vi "data_load_display_trend_fft_mea_coll_pred_v6.vi"() -> ()   [LabVIEW 2020]
uses:
  <vilib>/Utility/file.llb/Read Delimited Spreadsheet (DBL).vi
panel:
  out "truth vs prediction vs error":dbl[][](graph)
  out "Input vs prediction":dbl[][](graph)
  out "Time vs Acceleration ( Input learning length)":cluster{dbl[], dbl[]}[](graph)
  out "truth vs prediction":dbl[][](graph)
  out "Spectrum plot 2":cluster{i32, dbl, "spectrum out":dbl[]}(graph)
  out "Frequency Interval: delta(f) 2":dbl
  out "xf (frequency) 2":dbl[](array[numeric])
  out "size(s) 2":i32
  out "df (Hz) 2":dbl
  out "ploted signal from each selected frequency 2":dbl[][](graph)
  out "phase 3":dbl[](array[numeric])
  out "magnitude 3":dbl[](array[numeric])
  out "Time vs Acceleration graph(whole data)":cluster{"all rows":dbl[], "all rows":dbl[]}(graph)
  out "Acceleration 2":dbl[](array[numeric])
  out "time 2":dbl[](array[numeric])
  out "array w/ subset deleted 2":dbl[][](array[numeric])
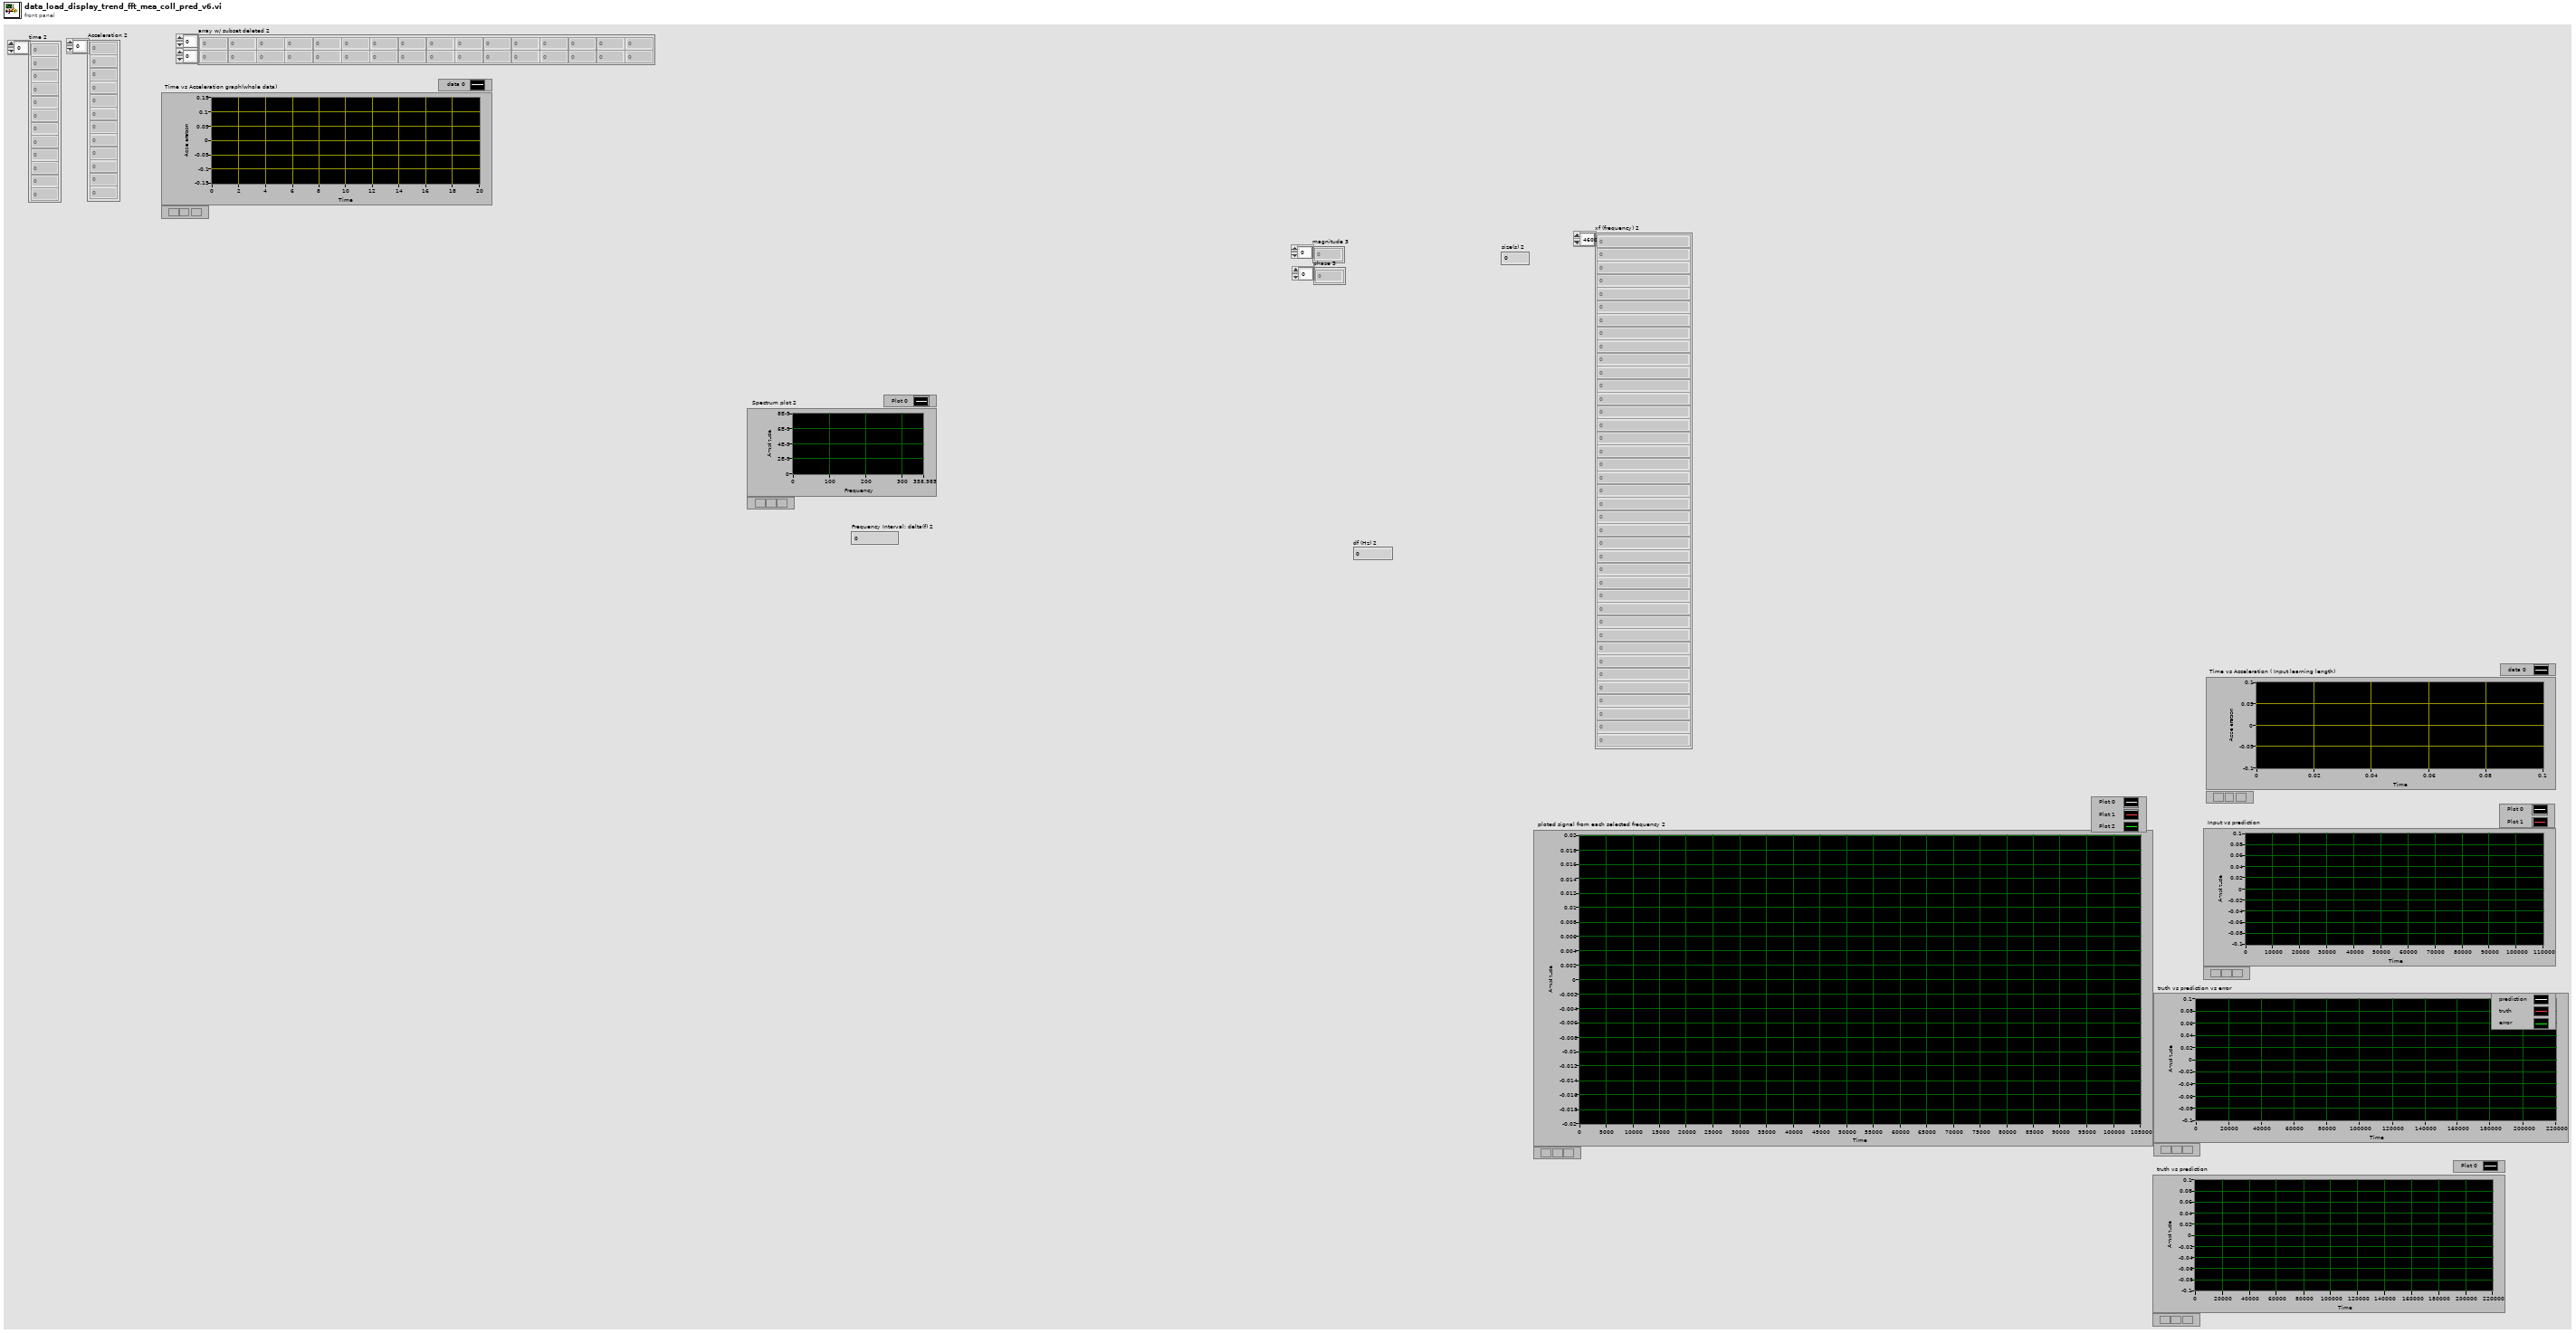
[diagram p1: front panel]
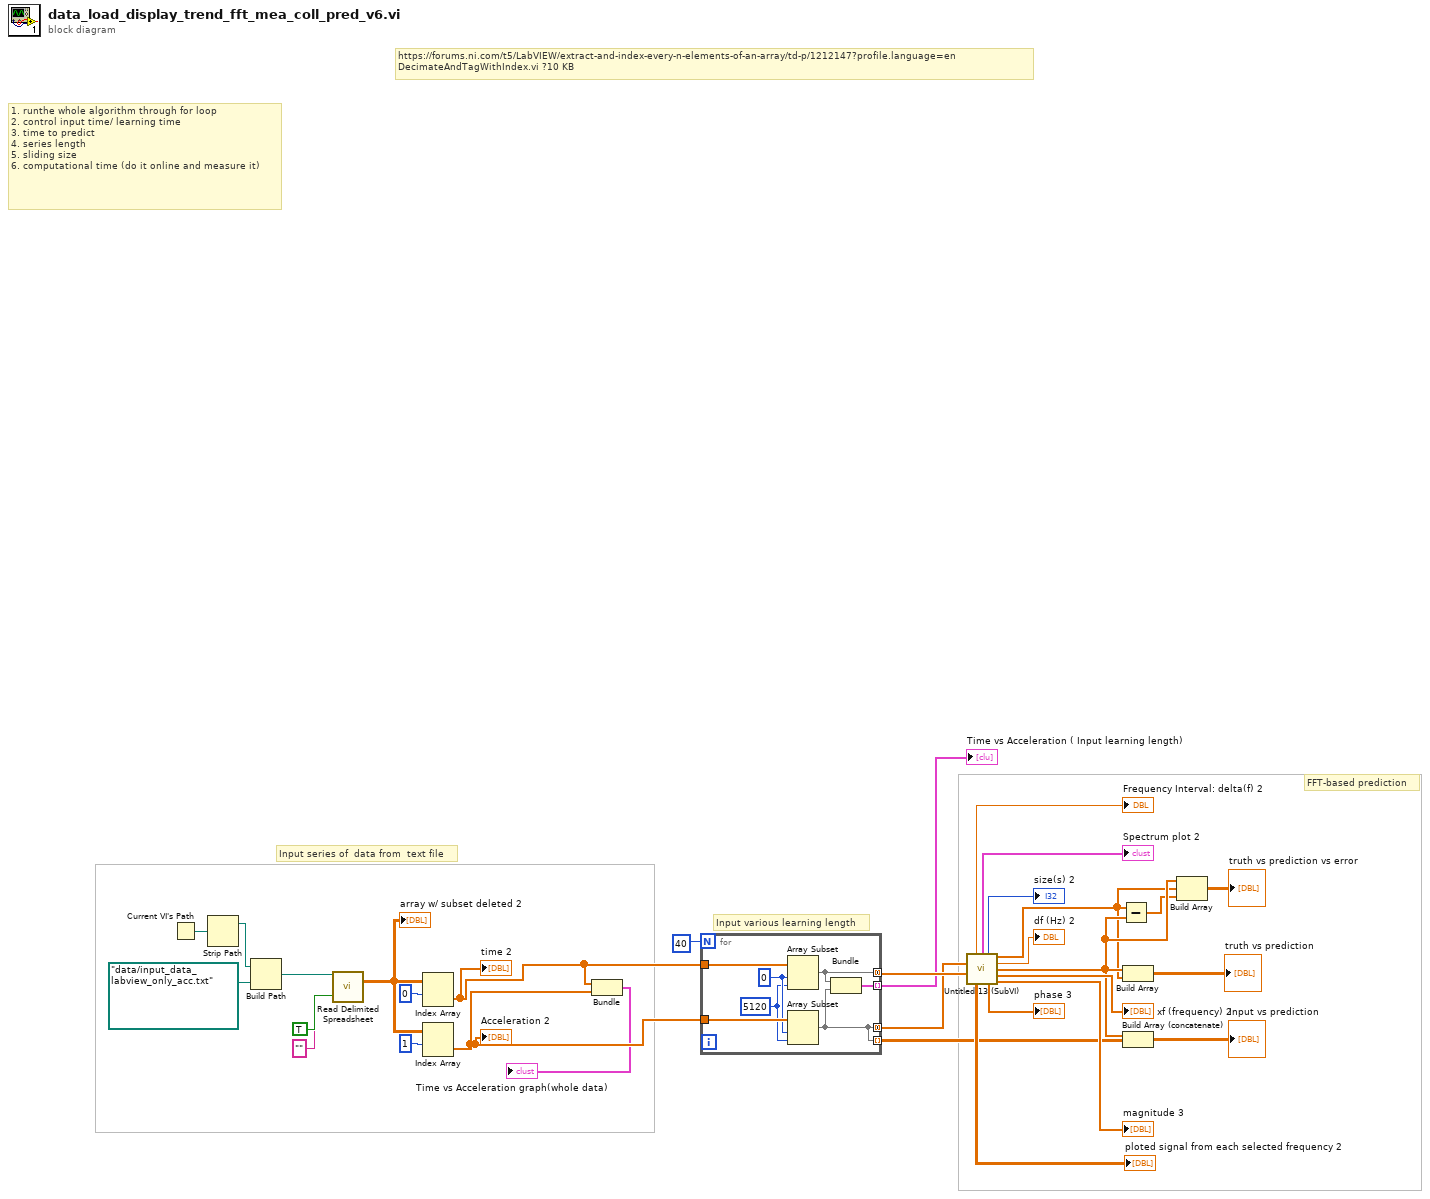
[diagram p0: block diagram]
diagram:
  # "Input series of  data from  text file"
  # "Input various learning length"
  # "FFT-based prediction"
  # "1. runthe whole algorithm through for loop \n2. control input time/ learning time\n3. time to predict\n4. series length\n5. sliding size\n6. computational time (do it online and measure it)"
  # "https://forums.ni.com/t5/LabVIEW/extract-and-index-every-n-elements-of-an-array/td-p/1212147?profile.language=en\nDecimateAndTagWithIndex.vi ?10 KB"
  n1 = Current VI's Path() -> (path=w29:path)
  n2 = Strip Path(path=w29) -> (stripped path=w30:path)  [unwired: 1 out]
  n3 = Build Path(base path=w30, name or relative path=path "data/input_data_labview_only_acc.txt") -> (appended path=w31:path)
  n4 = call-poly <vilib>:"Read Delimited Spreadsheet.vi"("file path (dialog if empty)"=w31, "transpose? (F)"=TRUE, "delimiter (\\t)"="" ("delimiter (\\t)")) -> ("all rows"=w28:dbl[][])  [unwired: 7 in, 5 out]
  "array w/ subset deleted 2" <- w28
  n5 = Index Array(array=w28, index (row)=0) -> (element=w13:dbl[])  [unwired: 1 in]
  "time 2" <- w13
  n6 = Index Array(array=w28, index (row)=1) -> (element=w11:dbl[])  [unwired: 1 in]
  "Acceleration 2" <- w11
  n7 = Bundle("all rows"=w13, "all rows"=w11) -> (→"Time vs Acceleration graph(whole data)":cluster{"all rows":dbl[], "all rows":dbl[]})  [unwired: 1 in]
  n8 = for {
    N: 40 -> [_]
    tunnel: w13 -> [w38]
    tunnel: [w35] -> w10 mode=concatenating
    tunnel: w11 -> [w37]
    tunnel: [w33] -> w9 mode=concatenating
    tunnel: [w34] -> w8 mode=indexing
    tunnel: [w33] -> w7 mode=indexing
    w36 = 0
    w32 = 5120 ("length")
    n9 = Array Subset(array=w38, index=w36, length=w32) -> (w35:dbl[])
    n10 = Array Subset(array=w37, index=w36, length=w32) -> (w33:dbl[])
    n11 = Bundle(w35, w33) -> (w34:cluster{dbl[], dbl[]})  [unwired: 1 in]
  }
  "Time vs Acceleration ( Input learning length)" <- w8
  n12 = call "Untitled 13 (SubVI).vi"("time"=w10, "acceleration"=w9) -> ("Frequency Interval: delta(f)"=→"Frequency Interval: delta(f) 2":dbl, "Spectrum plot"=→"Spectrum plot 2":cluster{i32, dbl, "spectrum out":dbl[]}, "size(s)"=→"size(s) 2":i32, "all rows"=w4:dbl[], "df (Hz)"=→"df (Hz) 2":dbl, "Array"=w5:dbl[], "xf (frequency)"=→"xf (frequency) 2":dbl[], "ploted signal from each selected frequency"=→"ploted signal from each selected frequency 2":dbl[][], "phase 2"=→"phase 3":dbl[], "magnitude 2"=→"magnitude 3":dbl[])  [unwired: 4 in]
  n13 = Subtract(x=w4, y=w5) -> (x-y=w3:dbl[])
  n14 = Build Array(w5, w4) -> (→"truth vs prediction":dbl[][])
  n15 = Build Array (concatenate)(w5, w7) -> (→"Input vs prediction":dbl[][])
  n16 = Build Array(w5, w4, w3) -> (→"truth vs prediction vs error":dbl[][])
